vi "backproject-master.vi"(9 "Image Properties":T1, 10 "Backproject Input":T3, 11 "Queue in":refnum<queue>) -> (1 "Selector":dbl, 2 "Projections":T2[](array[typedef]), 3 "Queue out":refnum<queue>)   [LabVIEW 2013]
uses:
  backproject_input.ctl
  bp_work_unit.ctl
  tags_cluster.ctl
  imagereconstruction/x64/Debug/labviewdll.dll
panel:
  in  "backproject work unit":T2
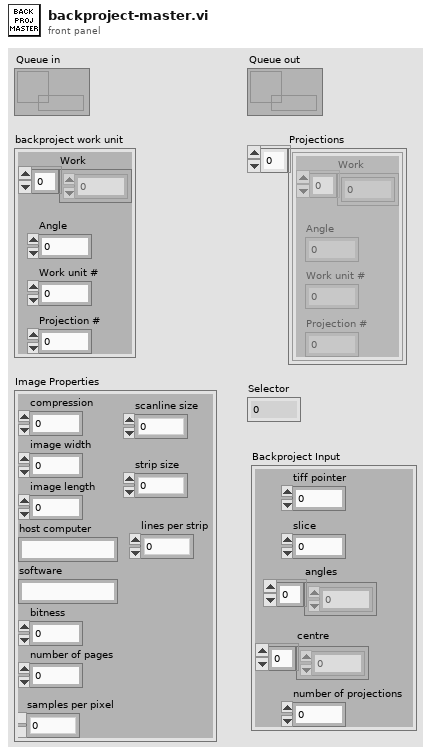
[diagram p1: front panel]
types:
  T1 = typedef "tags_cluster.ctl" = cluster{"compression":i32, "image width":i32, "image length":i32, "host computer":string, "software":string, "bitness":i32, "number of pages":i32, "samples per pixel":i32, "scanline size":i32, "strip size":i32, "lines per strip":i32}
  T2 = typedef "bp_work_unit.ctl" = cluster{"Work":u8[], "Angle":dbl, "Work unit #":i32, "Projection #":i32}
  T3 = typedef "backproject_input.ctl" = cluster{"tiff pointer":i64, "slice":u32, "angles":dbl[], "centre":i32[], "number of projections":u32}
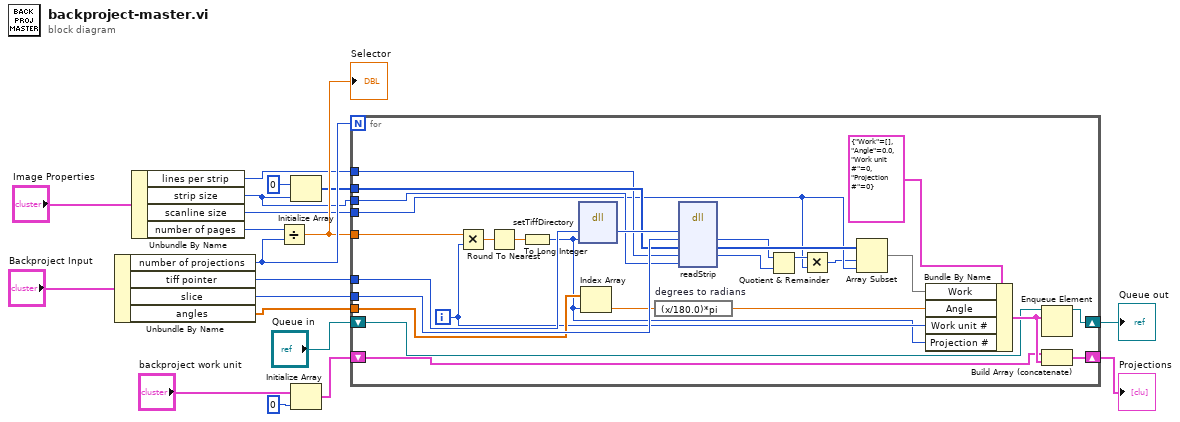
[diagram p0: block diagram]
diagram:
  n1 = Unbundle By Name("Backproject Input") -> ("number of projections"=w19:u32, "tiff pointer"=w15:i64, "slice"=w16:u32, "angles"=w17:dbl[])
  n2 = Unbundle By Name("Image Properties") -> ("lines per strip"=w3:i32, "strip size"=w5:i32, "scanline size"=w4:i32, "number of pages"=w18:i32)
  n3 = Divide(x=w18, y=w19) -> (x/y=w6:dbl)
  "Selector" <- w6
  n4 = Initialize Array(u8 0 ("element"), w5) -> (w2:u8[])
  n5 = Initialize Array("backproject work unit", 0 ("dimension size")) -> (w8:T2[])
  n6 = for {
    N: w19 -> [_]
    tunnel: w6 -> [w46]
    tunnel: w15 -> [w45]
    tunnel: w16 -> [w43]
    tunnel: w2 -> [w42]
    tunnel: w3 -> [w41]
    tunnel: w5 -> [w40]
    tunnel: w17 -> [w39]
    tunnel: w4 -> [w33]
    shift-right: [w25] -> w10
    shift-left: w8 -> [w26]
    shift-right: [w22] -> w12
    shift-left: "Queue in" -> [w23]
    i -> [w31]
    n7 = Multiply(x=w46, y=w31) -> (x*y=w29:dbl)
    n8 = Round To Nearest(number=w29) -> (nearest integer value=w28:dbl)
    n9 = To Long Integer(number=w28) -> (32bit integer=w24:i32)
    n10 = dll-call lib="D:/work/uni/FYP/reconrepo/imagereconstruction/x64/Debug/labviewdll.dll" fn="setTiffDirectory"("tiff"=w45, "directory"=w24) -> ("tiff"=w44:i64)  [unwired: 5 in, 2 out]
    n11 = Index Array(array=w39, index=w24) -> (element=w21:dbl)
    n12 = expression code="(x/180.0)*pi" "degrees to radians"(w21) -> (w20:dbl)
    n13 = dll-call lib="D:/work/uni/FYP/reconrepo/imagereconstruction/x64/Debug/labviewdll.dll" fn="readStrip"("tiff"=w44, "slice"=w43, "strip"=w42, "lines per strip"=w41, "strip size"=w40) -> ("slice"=w36:i32, "strip"=w38:u8[], "lines per strip"=w35:i32)  [unwired: 6 in, 2 out]
    n14 = Quotient & Remainder(x=w36, y=w35) -> (x-y*floor(x/y)=w34:i32)  [unwired: 1 out]
    n15 = Multiply(x=w34, y=w33) -> (x*y=w32:i32)
    n16 = Array Subset(array=w38, index=w32, length=w33) -> (w37:u8[])
    n17 = Bundle By Name(cluster=T2 {"Work"=[], "Angle"=0.0, "Work unit #"=0, "Projection #"=0} ("backproject work unit"), "Work"=w37, "Angle"=w20, "Work unit #"=w31, "Projection #"=w24) -> (w27:T2)
    n18 = Enqueue Element(queue=w23, element=w27) -> (queue out=w22:refnum<queue>)  [unwired: 2 in, 2 out]
    n19 = Build Array (concatenate)(w26, w27) -> (w25:T2[])
  }
  "Queue out" <- w12
  "Projections" <- w10
